vi "Log Debug.vi"(8 "error in (no error)":errorcluster, 10 "Message":string, 11 "Logging In":refnum<class "Logging.lvclass">) -> (0 "error out":errorcluster, 3 "Logging Out":refnum<class "Logging.lvclass">)   [LabVIEW 2020, in "Logging.lvclass"]
doc: "Enter a debug-level message into the system log. \nDebug level means detailed information, typically of interest only when diagnosing problems."
uses:
  Logging.lvclass
  Protected/Level.ctl
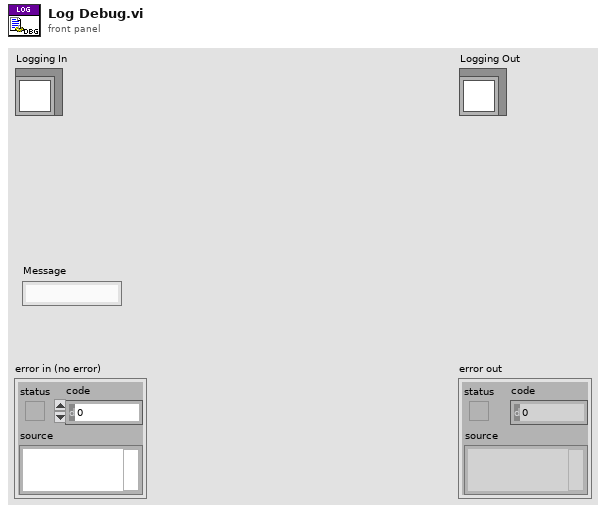
[diagram p1: front panel]
types:
  T1 = typedef "Logging.lvclass/Level.ctl" = enum16{"DEBUG", "INFO", "WARNING", "ERROR", "CRITICAL"}
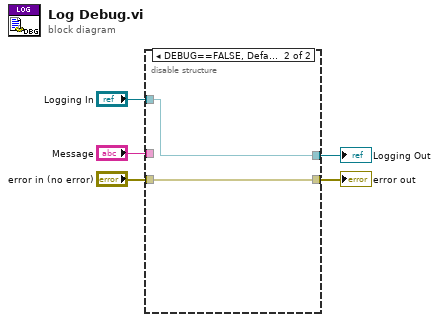
[diagram p0: block diagram]
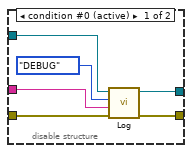
[diagram p2: hidden frame]
diagram:
  n1 = disable-structure shown="DEBUG==FALSE, Default" {
    disable-tunnel: "error in (no error)" -> [w11 w12]
    disable-tunnel: [w10 w12] -> w4
    disable-tunnel: "Logging In" -> [w9 w13]
    disable-tunnel: [w8 w13] -> w2
    disable-tunnel: "Message" -> [w7 _]
    frame condition #0 (active) {
      n2 = call-dynamic "Log.vi"("error in (no error)"=w11, "Message"=w7, "Level"=Level."DEBUG", "Logging In"=w9) -> ("error out"=w10:errorcluster, "Logging Out"=w8:refnum<class "Logging.lvclass">)  [unwired: 6 in]
    }
    frame condition #1 {
    }
  }
  "error out" <- w4
  "Logging Out" <- w2
